vi "IsEmpty.vi"(8 "error in (no error)":errorcluster caption="错误输入（无错误）", 11 "Point输入":refnum<class "Point.lvclass">) -> (0 "error out":errorcluster caption="错误输出", 2 "IsEmpty":bool, 3 "Point输出":refnum<class "Point.lvclass">)   [LabVIEW 2011, in "Point.lvclass"]
uses:
  Point.lvclass
  Point.lvclass/Point.ctl
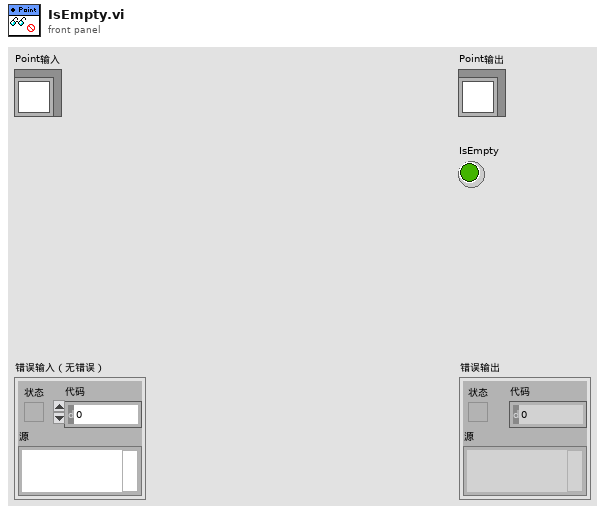
[diagram p1: front panel]
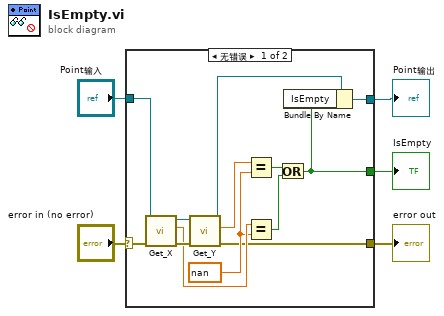
[diagram p0: block diagram]
diagram:
  n1 = case shown="无错误" "error in (no error)" {
    selector: "error in (no error)" -> [w15 w19]
    tunnel: [w6 w19] -> w4
    tunnel: [w7 w20] -> w2
    tunnel: "Point输入" -> [w18 w20]
    tunnel: [w8 _] -> w1
    frame No Error {
      w12 = nan ("y")
      n2 = call "Get_X.vi"("error in (no error)"=w15, "Point输入"=w18) -> ("error out"=w16:errorcluster, "X"=w14:dbl, "Point输出"=w17:refnum<class "Point.lvclass">)  [unwired: 7 in]
      n3 = call "Get_Y.vi"("error in (no error)"=w16, "Point输入"=w17) -> ("error out"=w6:errorcluster, "Y"=w13:dbl, "Point输出"=w9:refnum<class "Point.lvclass">)  [unwired: 7 in]
      n4 = Equal?(x=w13, y=w12) -> (x = y?=w11:bool)
      n5 = Equal?(x=w14, y=w12) -> (x = y?=w10:bool)
      n6 = Or(x=w11, y=w10) -> (x .or. y?=w8:bool)
      n7 = Bundle By Name(cluster=w9, "IsEmpty"=w8) -> (w7:refnum<class "Point.lvclass">)
    }
    frame Error {
    }
  }
  "error out" <- w4
  "Point输出" <- w2
  "IsEmpty" <- w1
